vi "open.vi"(8 "error in (no error)":errorcluster) -> (0 "error out":errorcluster, 3 "rethinkdb out":refnum<class "RethinkDB.lvclass">)   [LabVIEW 2017, in "rethinkdb.lvlib" / "RethinkDB.lvclass"]
uses:
  RethinkDB.lvclass
  connection.ctl
  RethinkDB.lvclass/RethinkDB.ctl
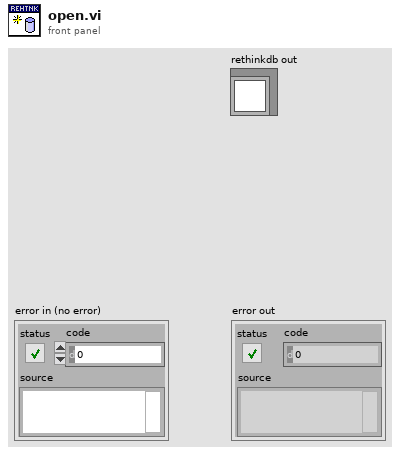
[diagram p1: front panel]
types:
  T1 = typedef "rethinkdb.lvlib/RethinkDB.lvclass/connection.ctl" = cluster{"host":string, "port":u16, "ms_timeout":i32, "conn":refnum<k5>, "auth_key":string}
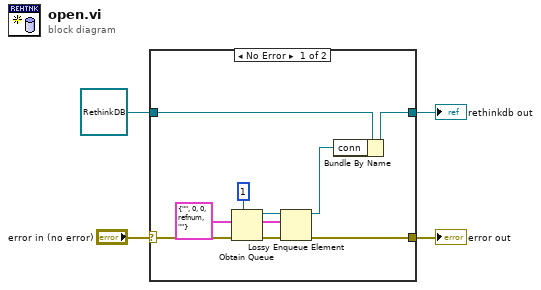
[diagram p0: block diagram]
diagram:
  n1 = case shown="No Error" "error in (no error)" {
    selector: "error in (no error)" -> [w10 w15]
    tunnel: [w6 w14] -> w4
    tunnel: [w9 w15] -> w2
    tunnel: refnum<class "RethinkDB.lvclass"> refnum ("rethinkdb.lvlib:rethinkdb") -> [w7 w14]
    frame No Error {
      w8 = T1 {"host"="", "port"=0, "ms_timeout"=0, "conn"=refnum, "auth_key"=""} ("connection")
      n2 = Obtain Queue(max queue size (-1, unlimited)=1, element data type=w8, error in (no error)=w10) -> (queue out=w12:refnum<queue>, error out=w11:errorcluster)  [unwired: 2 in, 1 out]
      n3 = Lossy Enqueue Element(queue=w12, element=w8, error in (no error)=w11) -> (queue out=w5:refnum<queue>, error out=w9:errorcluster)  [unwired: 2 out]
      n4 = Bundle By Name(cluster=w7, "conn"=w5) -> (w6:refnum<class "RethinkDB.lvclass">)
    }
    frame Error {
    }
  }
  "error out" <- w2
  "rethinkdb out" <- w4
